vi "dfd_FXP Rational Simu.vi"(0 "signal in":i64[](array[numeric]), 2 "PROD2SUM":i16, 3 "init?":bool, 5 "L":i32, 7 "M":i32, 9 "coef":i64[](array[numeric]), 11 "FXPMRateSimState in":T1, 12 "#taps per phase":i32) -> (4 "signal out":i64[](array[numeric]), 15 "FXPMRateSimState out":T1)   [LabVIEW 2017, in "NI_DigFilter_FXP.lvlib"]
uses:
  <vilib>/addons/Digital Filter Design/NI_DigFilter_FXP.lvlib
  <vilib>/addons/Digital Filter Design/_Objects.llb/dfd_FXP MRate Simu State.ctl
  <vilib>/addons/Digital Filter Design/_Objects.llb/dfd_Integer I160.ctl
  <vilib>/addons/Digital Filter Design/_Objects.llb/dfd_Index Config.ctl
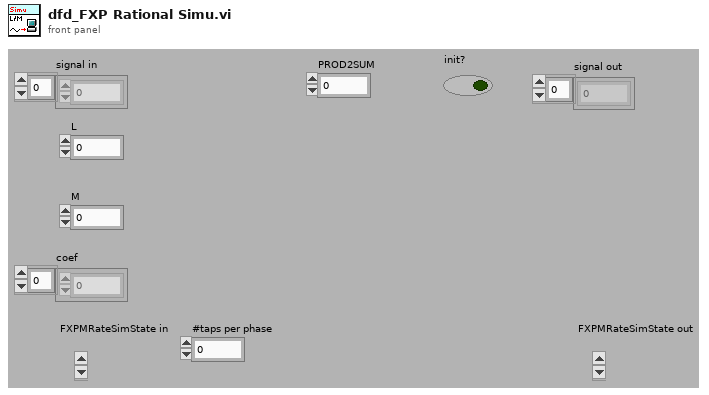
[diagram p1: front panel]
types:
  T1 = typedef "dfd_FXP MRate Simu State.ctl" = cluster{"acc1":T2[], "acc2":T2[], "FIR state":i64[], "next phase":i32}
  T2 = typedef "dfd_Integer I160.ctl" = cluster{"Hi [I32]":i32, "Lo3 [U32]":u32, "Lo2 [U32]":u32, "Lo1 [U32]":u32, "Lo0 [U32]":u32}
  T3 = typedef "dfd_Index Config.ctl" = cluster{"start":i32, "stepsize":i32}
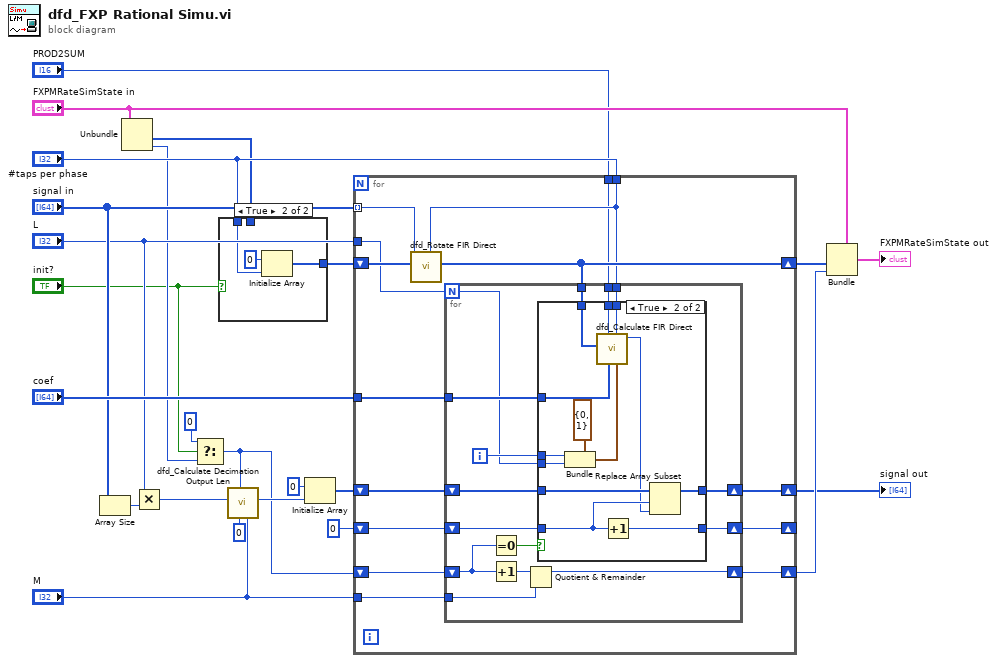
[diagram p0: block diagram]
diagram:
  n1 = Array Size(array="signal in") -> (size(s)=w22:i32)
  n2 = Unbundle("FXPMRateSimState in") -> ("FIR state"=w9:i64[], "next phase"=w10:i32)  [unwired: 2 out]
  n3 = Multiply(x="L", y=w22) -> (x*y=w20:i32)
  n4 = Select(t=0, s="init?", f=w10) -> (s? t:f=w8:i32)
  n5 = case shown="True" "init?" {
    tunnel: [w25 w27] -> w17
    tunnel: "#taps per phase" -> [_ w26]
    tunnel: w9 -> [w25 _]
    frame False {
    }
    frame True {
      n6 = Initialize Array(i64 0 ("element"), w26) -> (w27:i64[])
    }
  }
  n7 = call <vilib>:"dfd_Calculate Decimation Output Len.vi"("factor"="M", "output phase"=0, "current phase"=w8, "signal in len"=w20) -> ("signal out len"=w13:i32)  [unwired: 7 out]
  n8 = Initialize Array(i64 0 ("element"), w13) -> (w15:i64[])
  n9 = for {
    tunnel: "signal in" -> [w41] mode=indexing
    tunnel: "L" -> [w32]
    tunnel: "#taps per phase" -> [w30]
    shift-right: [w31] -> w6
    shift-left: w17 -> [w40]
    tunnel: "coef" -> [w42]
    shift-right: [w35] -> w1
    shift-left: w15 -> [w38]
    tunnel: "M" -> [w37]
    shift-right: [w33] -> w5
    shift-left: w8 -> [w39]
    shift-right: [w34] -> _
    shift-left: 0 -> [w36]
    tunnel: "PROD2SUM" -> [w29]
    n10 = call <vilib>:"dfd_Rotate FIR Direct.vi"("#taps per phase"=w30, "state in"=w40, "x"=w41) -> ("state out"=w31:i64[])  [unwired: 1 in, 7 out]
    n11 = for {
      N: w32 -> [w54]
      tunnel: w30 -> [w55]
      tunnel: w31 -> [w45]
      tunnel: w42 -> [w57]
      shift-right: [w50] -> w33
      shift-left: w39 -> [w44]
      shift-right: [w47] -> w35
      shift-left: w38 -> [w53]
      tunnel: w37 -> [w51]
      shift-right: [w48] -> w34
      shift-left: w36 -> [w49]
      tunnel: w29 -> [w43]
      i -> [w56]
      n12 = Equal To 0?(x=w44) -> (x = 0?=w46:bool)
      n13 = Increment(x=w44) -> (x+1=w52:i32)
      n14 = Quotient & Remainder(x=w52, y=w51) -> (x-y*floor(x/y)=w50:i32)  [unwired: 1 out]
      n15 = case shown="True" w46 {
        tunnel: w57 -> [_ w61]
        tunnel: w56 -> [_ w71]
        tunnel: w55 -> [_ w70]
        tunnel: w45 -> [_ w68]
        tunnel: w54 -> [_ w67]
        tunnel: w53 -> [w59 w66]
        tunnel: w49 -> [w58 w65]
        tunnel: [w58 w64] -> w48
        tunnel: [w59 w63] -> w47
        tunnel: w43 -> [_ w60]
        frame False {
        }
        frame True {
          n16 = Bundle(cluster=T3 {"start"=0, "stepsize"=1} ("state idx"), "start"=w71, "stepsize"=w67) -> (w69:T3)
          n17 = call <vilib>:"dfd_Calculate FIR Direct.vi"("coef idx"=w69, "#taps per phase"=w70, "coef"=w61, "fwl_diff"=w60, "state in"=w68) -> ("y"=w62:i64)  [unwired: 3 in, 3 out]
          n18 = Increment(x=w65) -> (x+1=w64:i32)
          n19 = Replace Array Subset(array=w66, new element=w62, index=w65) -> (w63:i64[])
        }
      }
    }
  }
  "signal out" <- w1
  n20 = Bundle(cluster="FXPMRateSimState in", "FIR state"=w6, "next phase"=w5) -> (→"FXPMRateSimState out":T1)  [unwired: 2 out]
